vi "Fct_Acquisition_Temperature.vi"(10 "Unité":enum32{"° C", "° F", "° K"}(ring), 11 "Tension":dbl) -> (0 "Test":dbl, 1 "Echelle Min":dbl, 2 "Echelle Max":dbl, 3 "Température":dbl)   [LabVIEW 2017]
doc: "Converti une tension en température selon la valeur de l'unité.\nESIGELEC\n5 Octobre\nBenoit Mangeard\n.............................."
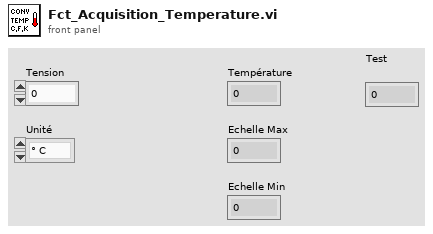
[diagram p1: front panel]
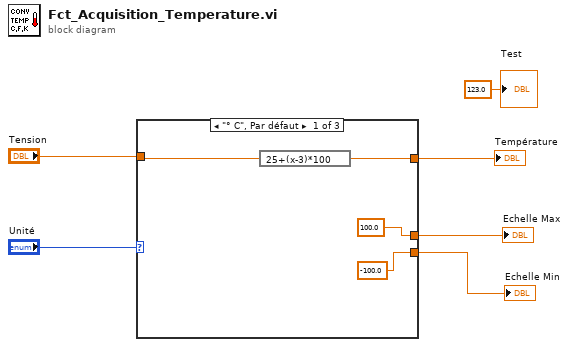
[diagram p0: block diagram]
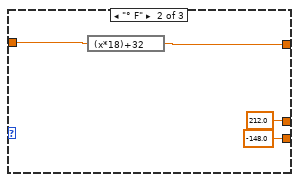
[diagram p2: hidden frame]
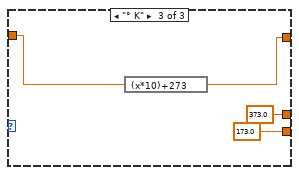
[diagram p3: hidden frame]
diagram:
  n1 = case shown="\"° C\", Par défaut" "Unité" {
    tunnel: "Tension" -> [w10 w14 w18]
    tunnel: [w9 w13 w17] -> w3
    tunnel: [100.0 212.0 373.0] -> w4
    tunnel: [-100.0 -148.0 173.0] -> w5
    frame "° C", Default {
      n2 = expression code="25+(x-3)*100"(w10) -> (w9:dbl)
    }
    frame "° F" {
      n3 = expression code="(x*18)+32"(w14) -> (w13:dbl)
    }
    frame "° K" {
      n4 = expression code="(x*10)+273"(w18) -> (w17:dbl)
    }
  }
  "Echelle Min" <- w5
  "Echelle Max" <- w4
  "Température" <- w3
  "Test" <- 123.0 ("Test")
